vi "SendWelcome.vi"(8 "error in (no error)":errorcluster, 11 "TCP_Server_Connection_Handler in":refnum<class "TCP_Server_Connection_Handler.lvclass">) -> (0 "error out":errorcluster, 3 "TCP_Server_Connection_Handler out":refnum<class "TCP_Server_Connection_Handler.lvclass">)   [LabVIEW 2023, in "TCP_Server_Connection_Handler.lvlib" / "TCP_Server_Connection_Handler.lvclass"]
uses:
  TCP_Server_Connection_Handler.lvclass
  TCP_Server_Connection_Handler.lvclass/TCP_Server_Connection_Handler.ctl
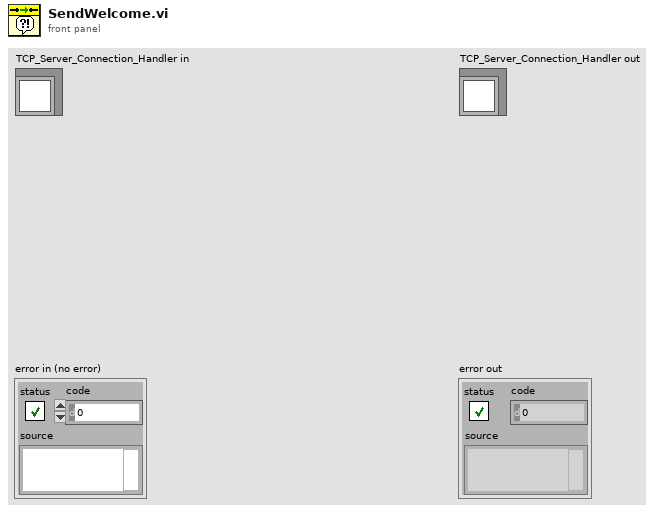
[diagram p1: front panel]
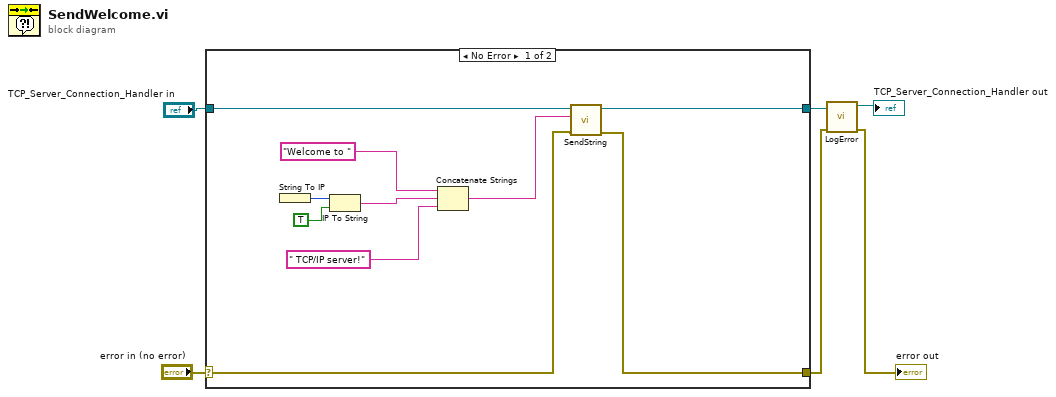
[diagram p0: block diagram]
diagram:
  n1 = case shown="No Error" "error in (no error)" {
    selector: "error in (no error)" -> [w8 w18]
    tunnel: [w7 w18] -> w2
    tunnel: [w10 w17] -> w4
    tunnel: "TCP_Server_Connection_Handler in" -> [w11 w17]
    frame No Error {
      n2 = String To IP() -> (0:w16:u32)  [unwired: 1 in]
      n3 = IP To String(1:TRUE ("dot notation? (F)"), 2:w16) -> (0:w13:string)
      n4 = Concatenate Strings("Welcome to ", w13, " TCP/IP server!" ("string")) -> (w9:string)
      n5 = call "SendString.vi"("error in (no error)"=w8, "Message"=w9, "TCP_Server_Connection_Handler in"=w11) -> ("error out"=w7:errorcluster, "TCP_Server_Connection_Handler out"=w10:refnum<class "TCP_Server_Connection_Handler.lvclass">)  [unwired: 7 in]
    }
    frame Error {
    }
  }
  n6 = call "LogError.vi"("error in (no error)"=w2, "TCP_Server_Connection_Handler in"=w4) -> ("error out"=→"error out":errorcluster, "TCP_Server_Connection_Handler out"=→"TCP_Server_Connection_Handler out":refnum<class "TCP_Server_Connection_Handler.lvclass">)  [unwired: 8 in]
